vi "Generator sygnałów testowych1.vi"(2 "częstość pobierania\nserii próbek":dbl format="%.2f", 3 "liczba punktów\n      (1024)":i32, 4 "amplituda  szumów":dbl(knob)=50.0 scale=50.0..1000.0, 5 "amplituda":dbl(knob)=50.0 scale=50.0..1000.0, 6 "częstotliwość":dbl(knob)=50.0 scale=50.0..1000.0, 7 "typ sygnału":u16(ring)=1 items=["szum", "zewnętrzny", "sinus", "prostokąt", "trójkąt"]) -> (0 "czas pobierania\nserii próbek":dbl format="%.2f", 1 "Sygnał wyjściowy":dbl[](array[numeric]) format="%.2f")   [LabVIEW 2020]
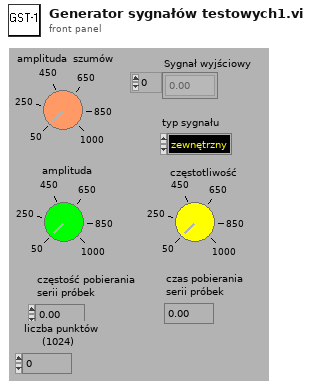
[diagram p1: front panel]
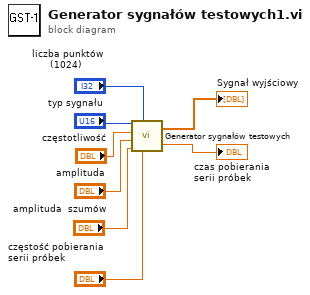
[diagram p0: block diagram]
diagram:
  n1 = call "Generator sygnałów testowych.vi"("częstotliwość\nakwizycji próbek"="częstość pobierania\nserii próbek", "liczba punktów\n      (1024)"="liczba punktów\n      (1024)", "amplituda szumów"="amplituda  szumów", "amplituda sygnału"="amplituda", "częstotliwość\n   sygnału"="częstotliwość", "rodzaj sygnału"="typ sygnału") -> ("czas akwizycji\n      próbek"=→"czas pobierania\nserii próbek":dbl, "sygnał wyjściowy"=→"Sygnał wyjściowy":dbl[])
